vi "Read Triggering.vi"(8 "error in (no error)":errorcluster, 11 "Ni-Scope Digitizer in":refnum<class "Ni-Scope Digitizer.lvclass">) -> (0 "error out":errorcluster, 2 "Triggering":enum16{"Reference", "Start"}(ring), 3 "Ni-Scope Digitizer out":refnum<class "Ni-Scope Digitizer.lvclass">)   [LabVIEW 2016, in "Ni-Scope Digitizer.lvclass"]
uses:
  Ni-Scope Digitizer.lvclass
  Ni-Scope Digitizer.lvclass/Ni-Scope Digitizer.ctl
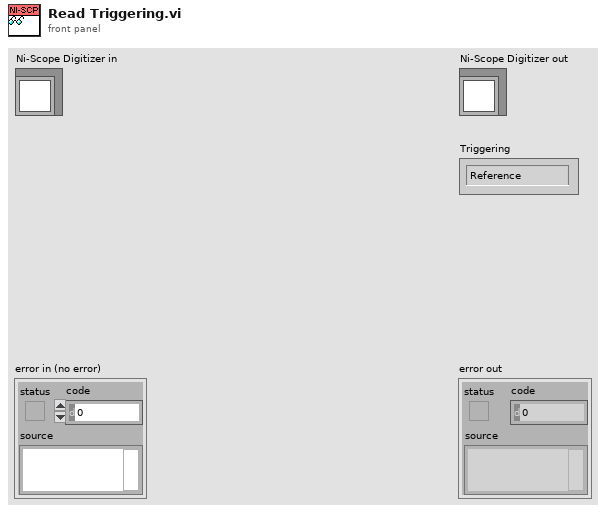
[diagram p1: front panel]
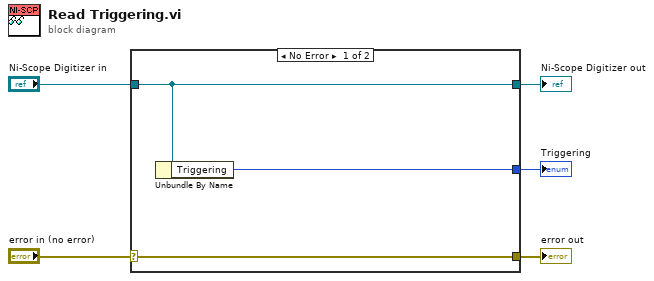
[diagram p0: block diagram]
diagram:
  n1 = case shown="No Error" "error in (no error)" {
    selector: "error in (no error)" -> [w8 w9]
    tunnel: [w8 w9] -> w4
    tunnel: [w7 w10] -> w2
    tunnel: "Ni-Scope Digitizer in" -> [w7 w10]
    tunnel: [w6 _] -> w1
    frame No Error {
      n2 = Unbundle By Name(w7) -> ("Triggering"=w6:enum16{"Reference", "Start"})
    }
    frame Error {
    }
  }
  "error out" <- w4
  "Ni-Scope Digitizer out" <- w2
  "Triggering" <- w1
